vi "NISE.remote.Read Register (Core).vi"(0 "SLSC Remote in":refnum<class "SLSC Interface.lvclass">, 1 "type":enum16{"U8", "U16", "U32", "U64"}(ring), 5 "device":refnum<k21>="$DefaultDevices", 7 "register address":u32 format="%.0x", 11 "error in (no error)":errorcluster) -> (4 "SLSC Remote out":refnum<class "SLSC Interface.lvclass">, 6 "device out":refnum<k21>, 8 "next register address":u32 format="%.0x", 10 "data out":u64 format="%.0x", 15 "error out":errorcluster)   [LabVIEW 2016, in "SLSC Interface.lvclass"]
uses:
  SLSC Interface Class/SLSC Interface.lvclass
  SLSC Interface Class/SLSC Interface.lvclass/SLSC Interface.ctl
  SLSC Interface Class/NISE.Read client handle.vi
  SLSC Interface Class/NISE.Read URL.vi
  <vilib>/NI/JSON Support for LabVIEW/JSON Data Classes/JSON Object/JSON Object.lvclass
  C:/Program Files (x86)/National Instruments/LabVIEW 2016/vi.lib/NI/JSON Support for LabVIEW/JSON Data Classes/JSON Datatype/JSON Null.lvclass
  SLSC Interface Class/NISE.Read session.vi
  <vilib>/NI/JSON Support for LabVIEW/JSON Data Classes/JSON Object/New JSON Object (Empty).vi
  <vilib>/NI/JSON Support for LabVIEW/JSON Data Classes/JSON Object/Insert Key Value Pair (Single String).vi
  <vilib>/NI/JSON Support for LabVIEW/JSON Data Classes/JSON Object/Insert Key Value Pair (Single Numeric).vi
  <vilib>/NI/NI JSONRPC Server Framework/Classes/Server/Format Client Request (Auto-Increment).vi
  <vilib>/httpClient/POSTBuffer.vi
  <vilib>/NI/NI JSONRPC Server Framework/Classes/Server/Parse Response (Object).vi
  <vilib>/NI/JSON Support for LabVIEW/JSON Data Classes/JSON Object/Get Value (Numeric Value).vi
  <vilib>/NI/NI JSONRPC Server Framework/Classes/Server/JSONRPC Server.lvclass
  <vilib>/httpClient/LabVIEWHTTPClient.lvlib
  <vilib>/NI/JSON Support for LabVIEW/JSON Data Classes/JSON Helper/JSON Helper.lvclass
  C:/Program Files (x86)/National Instruments/LabVIEW 2016/vi.lib/NI/JSON Support for LabVIEW/JSON Data Classes/JSON Structured Type/JSON Structure.lvclass
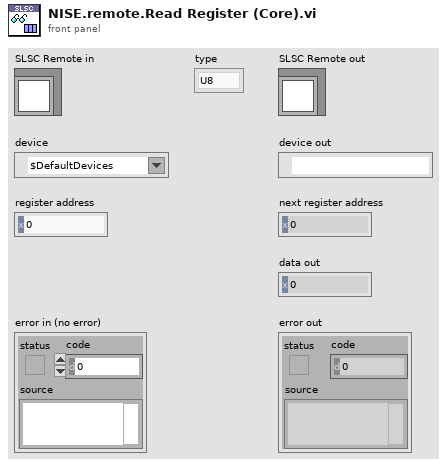
[diagram p1: front panel]
types:
  T1 = typedef "LabVIEWHTTPClient.lvlib/ClientHandle.ctl" = refnum<k1>
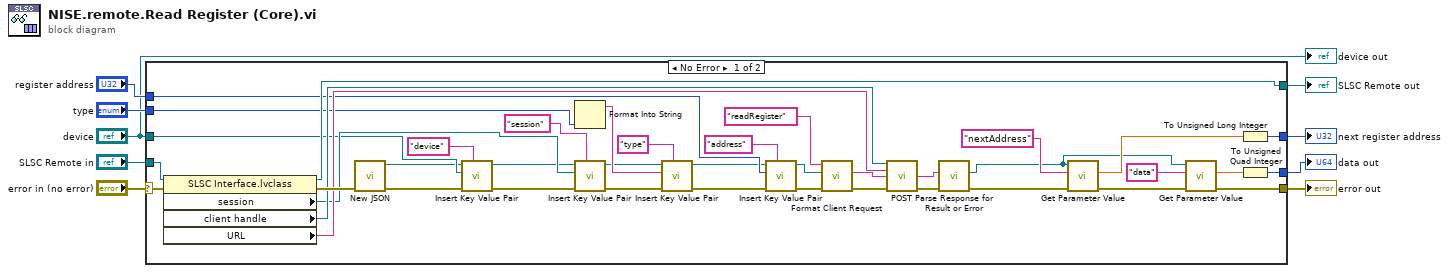
[diagram p0: block diagram]
diagram:
  n1 = case shown="No Error" "error in (no error)" {
    selector: "error in (no error)" -> [w47 w50]
    tunnel: "device" -> [w15 _]
    tunnel: "SLSC Remote in" -> [w49 w51]
    tunnel: [w48 w51] -> w4
    tunnel: [w32 w50] -> w3
    tunnel: "type" -> [w36 _]
    tunnel: "register address" -> [w18 _]
    tunnel: [w31 _] -> w2
    tunnel: [w29 _] -> w1
    frame No Error {
      n2 = property class="SLSC Interface.lvclass"(reference=w49, error in=w47) -> (reference out=w48:refnum<class "SLSC Interface.lvclass">, error out=w46:errorcluster, "session"=w16:refnum<k21>, "client handle"=w41:T1, "URL"=w40:string)
      n3 = call-poly <vilib>:"New JSON.vi"("error in (no error)"=w46) -> ("error out"=w45:errorcluster, "JSON Object out"=w14:refnum<class "JSON Object.lvclass">)  [unwired: 9 in]
      n4 = call-poly <vilib>:"Insert Key Value Pair.vi"("key"="device" ("Name"), "error in (no error)"=w45, "value"=w15, "JSON Object in"=w14) -> ("error out"=w44:errorcluster, "JSON Object out"=w13:refnum<class "JSON Object.lvclass">)  [unwired: 5 in, 1 out]
      n5 = Format Into String(w36) -> (resulting string=w17:string)  [unwired: 3 in, 1 out]
      n6 = call-poly <vilib>:"Insert Key Value Pair.vi"("key"="session" ("Name"), "error in (no error)"=w44, "value"=w16, "JSON Object in"=w13) -> ("error out"=w28:errorcluster, "JSON Object out"=w12:refnum<class "JSON Object.lvclass">)  [unwired: 5 in, 1 out]
      n7 = call-poly <vilib>:"Insert Key Value Pair.vi"("key"="type" ("Name"), "error in (no error)"=w28, "value"=w17, "JSON Object in"=w12) -> ("error out"=w27:errorcluster, "JSON Object out"=w11:refnum<class "JSON Object.lvclass">)  [unwired: 5 in, 1 out]
      n8 = call-poly <vilib>:"Insert Key Value Pair.vi"("key"="address" ("Name"), "error in (no error)"=w27, "value"=w18, "JSON Object in"=w11) -> ("error out"=w34:errorcluster, "JSON Object out"=w35:refnum<class "JSON Object.lvclass">)  [unwired: 5 in, 1 out]
      n9 = call-poly <vilib>:"Format Client Request.vi"("error in (no error)"=w34, "JSON in"=w35, "method"="readRegister") -> ("error out"=w39:errorcluster, "Request String"=w42:string)  [unwired: 7 in]
      n10 = call-poly <vilib>:"POST.vi"("client handle"=w41, "url"=w40, "buffer"=w42, "error in (no error)"=w39) -> ("body"=w38:string, "error out"=w37:errorcluster)  [unwired: 8 in, 2 out]
      n11 = call-poly <vilib>:"Parse Response for Result or Error.vi"("error in"=w37, "Response String In"=w38) -> ("error out"=w24:errorcluster, "JSON Array"=w10:refnum<class "JSON Object.lvclass">)  [unwired: 7 in, 1 out]
      n12 = call-poly <vilib>:"Get Parameter Value.vi"("error in (no error)"=w24, "key"="nextAddress" ("Parameter Name"), "JSON Object in"=w10) -> ("error out"=w33:errorcluster, "value"=w23:dbl)  [unwired: 7 in]
      n13 = call-poly <vilib>:"Get Parameter Value.vi"("error in (no error)"=w33, "key"="data" ("Parameter Name"), "JSON Object in"=w10) -> ("error out"=w32:errorcluster, "value"=w30:dbl)  [unwired: 7 in]
      n14 = To Unsigned Long Integer(number=w23) -> (unsigned 32bit integer=w31:u32)
      n15 = To Unsigned Quad Integer(1:w30) -> (0:w29:u64)
    }
    frame Error {
    }
  }
  "error out" <- w3
  "SLSC Remote out" <- w4
  "next register address" <- w2
  "data out" <- w1
  "device out" <- "device"
